vi "Top VI.vi"() -> ()   [LabVIEW 2018]
uses:
  <vilib>/addons/Modulation/niDMT.lvlib
panel:
  out "FALSE Subcarriers":i32
  out "Total Subcarriers":i32
  out "Total Bits":i32
  out "FALSE Bits":i32
  out "Constellation Graph":T1(graph)
  out "Waveform Chart":waveform(dbl)(graph)
  in  "QAM Complexity":T2(ring)
  in  "QAM Comparison":enum16{"MT Modulate", "Homebrew"}(ring)
  in  "Number of Symbols":i32=1
  in  "Samples/Symbol":i32=12
  in  "Symbol Rate":i32=1
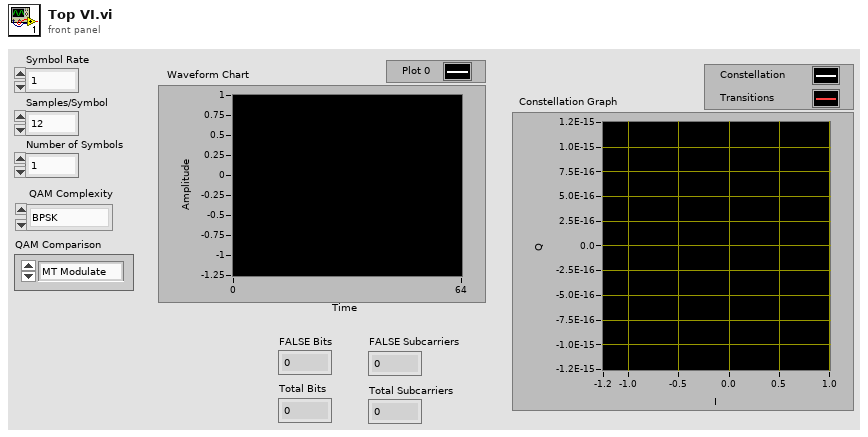
[diagram p1: front panel]
types:
  T1 = cluster{"Decimated Array":dbl[], "Decimated Array":dbl[]}[]
  T2 = enum16{"BPSK", "QPSK", "16-QAM", "64-QAM", "256-QAM"}
  T3 = typedef "niAMT.lvlib/Complex Data Waveform.ctl" = cluster{"t0":dbl, "dt":dbl, "Y":cdb[]}
  T4 = cluster{"constellation":dbl[], "oversampled data":dbl[]}[]
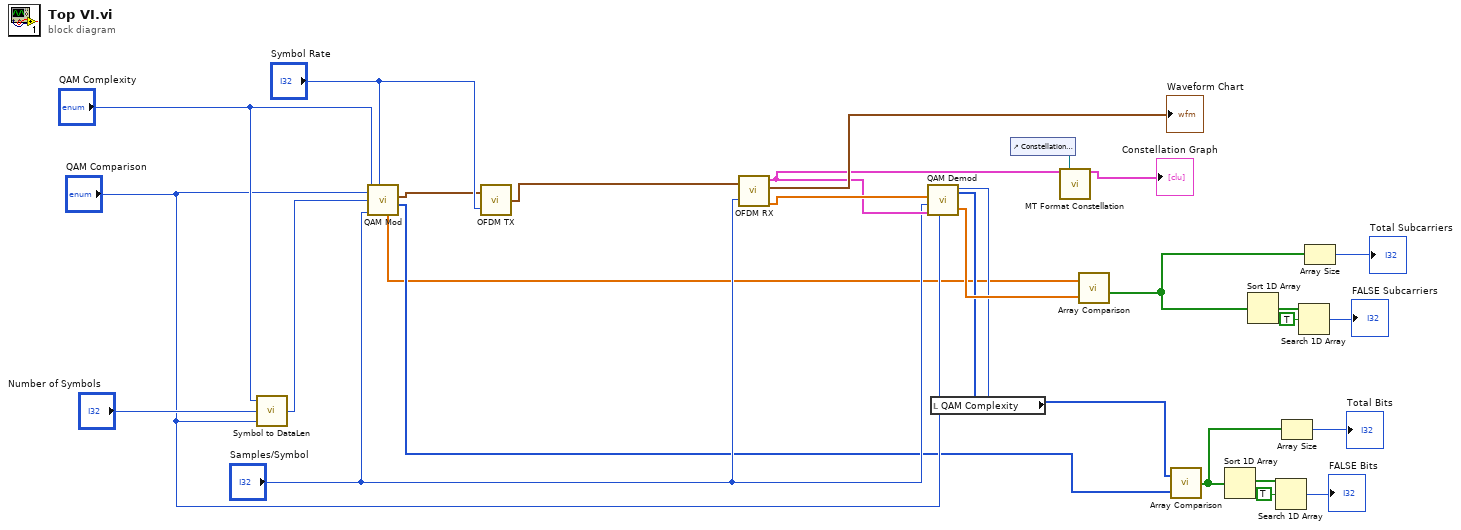
[diagram p0: block diagram]
diagram:
  n1 = call "Symbol to DataLen.vi"("QAM Comparison"="QAM Comparison", "Number of Symbols"="Number of Symbols", "QAM Complexity"="QAM Complexity") -> ("DataLen"=w5:i32)
  n2 = call "QAM Mod.vi"("Symbol Rate"="Symbol Rate", "Samples/Symbol"="Samples/Symbol", "DataLen"=w5, "QAM Comparison"="QAM Comparison", "QAM Complexity"="QAM Complexity") -> ("Bitstream (Reference)"=w2:i32[], "Waveform"=w3:waveform(cdb), "Data SCs (Reference)"=w1:cdb[])  [unwired: 2 out]
  n3 = call "OFDM TX.vi"("Symbol Rate"="Symbol Rate", "Waveform"=w3) -> ("TX Signal"=w24:waveform(cdb))
  n4 = call "OFDM RX.vi"("Waveform"=w24, "Samples/Symbol"="Samples/Symbol") -> ("Complex Waveform"=w20:T3, "Out - Waveform"=→"Waveform Chart":waveform(dbl), "Out  - Digital Subcarriers"=w21:cdb[])  [unwired: 1 out]
  n5 = local read "QAM Complexity"() -> (w25:T2)
  n6 = call "QAM Demod.vi"("QAM Complexity"=w25, "FFT"=w21, "Samples/Symbol"="Samples/Symbol", "input complex waveform"=w20, "QAM Comparison"="QAM Comparison") -> ("BitStream Out"=w19:i32[], "QAM Data Symbols"=w26:cdb[])
  n7 = control-ref of="Constellation Graph"() -> (w28:refnum<vi>)
  n8 = call <vilib>:"MT Format Constellation.vi"("waveform"=w20, "constellation reference"=w28) -> ("constellation graph"=→"Constellation Graph":T4)  [unwired: 3 in, 10 out]
  n9 = call "Array Comparison.vi"("Bit STream 2"=w26, "Bit Stream 1"=w1) -> ("Bit Stream Comparison"=w9:bool[])
  n10 = call "Array Comparison.vi"("Bit STream 2"=w2, "Bit Stream 1"=w19) -> ("Bit Stream Comparison"=w14:bool[])
  n11 = Sort 1D Array(array=w14) -> (sorted array=w17:bool[])
  n12 = Sort 1D Array(array=w9) -> (sorted array=w11:bool[])
  n13 = Search 1D Array(1D array=w17, element=TRUE) -> (index of element=→"FALSE Bits":i32)  [unwired: 1 in]
  n14 = Array Size(array=w14) -> (size(s)=→"Total Bits":i32)
  n15 = Search 1D Array(1D array=w11, element=TRUE) -> (index of element=→"FALSE Subcarriers":i32)  [unwired: 1 in]
  n16 = Array Size(array=w9) -> (size(s)=→"Total Subcarriers":i32)
